vi "FTW-Container-Object-Element-Delete.vi"(0 "FTW-Container In":refnum<class "FTW-Container.lvclass">, 5 "Element Name":string, 11 "error in":errorcluster) -> (4 "FTW-Container Out":refnum<class "FTW-Container.lvclass">, 8 "Found":bool, 15 "error out":errorcluster)   [LabVIEW 2015, in "FTW-Container.lvclass"]
uses:
  FTW-Container.lvclass
  FTW-Container.lvclass/FTW-Container.ctl
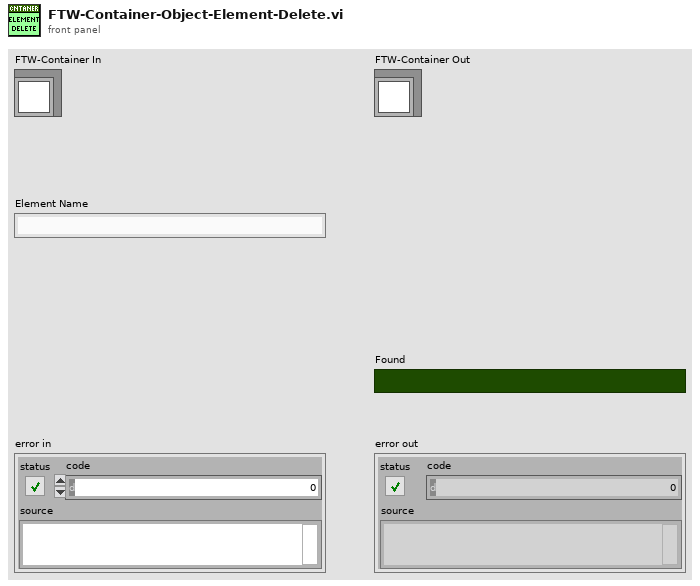
[diagram p1: front panel]
types:
  T1 = typedef "FTW-Container.lvclass/FTW-Container-Object.ctl" = cluster{"Names":string[], "Values":variant[]}
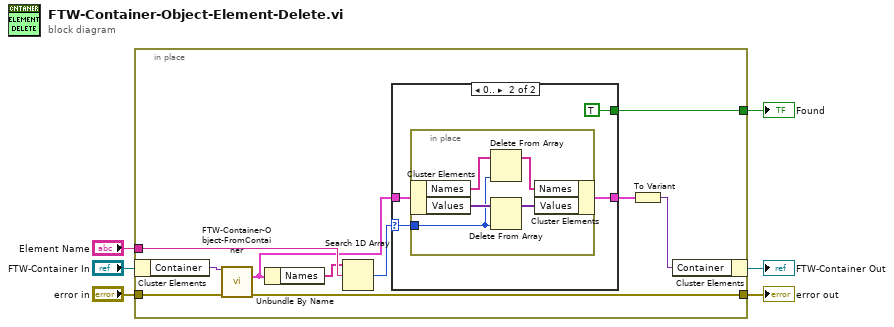
[diagram p0: block diagram]
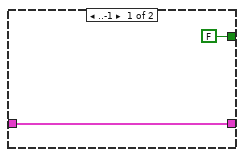
[diagram p2: hidden frame]
diagram:
  n1 = in-place {
    in-place-border: "error in" -> [w16]
    in-place-border: [w13] -> w3
    in-place-border: [w10] -> w2
    in-place-border: "Element Name" -> [w14]
    n2 = in-place-cluster #1("FTW-Container In") -> ("Container"=w15:variant)
    n3 = call "FTW-Container-Object-FromContainer.vi"("FTW-Container In"=w15, "error in"=w16) -> (6:w9:T1, "error out"=w13:errorcluster)  [unwired: 12 in]
    n4 = Unbundle By Name(w9) -> ("Names"=w12:string[])
    n5 = Search 1D Array(1D array=w12, element=w14) -> (index of element=w11:i32)  [unwired: 1 in]
    n6 = case shown="0.." w11 {
      selector: w11 -> [_ w19]
      tunnel: [FALSE TRUE] -> w10
      tunnel: w9 -> [w17 w21]
      tunnel: [w17 w20] -> w8
      frame ..-1 {
      }
      frame 0.. {
        n7 = in-place {
          in-place-border: w19 -> [w23]
          n8 = in-place-cluster #2(w21) -> ("Names"=w27:string[], "Values"=w25:variant[])
          n9 = Delete From Array(array=w27, index=w23) -> (array with subset deleted=w26:string[])  [unwired: 1 in, 1 out]
          n10 = Delete From Array(array=w25, index=w23) -> (array with subset deleted=w24:variant[])  [unwired: 1 in, 1 out]
          n11 = in-place-cluster #2("Names"=w26, "Values"=w24) -> (w20:T1)
        }
      }
    }
    n12 = To Variant(anything=w8) -> (Variant=w7:variant)
    n13 = in-place-cluster #1("Container"=w7) -> (→"FTW-Container Out":refnum<class "FTW-Container.lvclass">)
  }
  "error out" <- w3
  "Found" <- w2
